vi "PhotonUtils_EstimateCameraToTargetTrans.vi"(10 "Yaw":T2={"VALUE"=0.0, "COS"=1.0, "SIN"=0.0} {"SIN" format="%13.4f"; "COS" format="%13.4f"; "VALUE" format="%13.4f"}, 11 "TargetDistance_Meters":dbl) -> (3 "CameraToTarget":T1 {"Y" format="%14.3f"; "X" format="%14.3f"})   [LabVIEW 2020, in "PhotonVisionLib.lvlib"]
doc: "Estimate the Translation2d of the target relative to the camera.\n \nInputs: \n - TargetDistance_Meters -- The distance to the target in meters.\n - Yaw -- The observed yaw of the target.\n\nOutputs:\n - CameraToTarget -- The target's camera-relative translation."
uses:
  PhotonVisionLib.lvlib
  <vilib>/Rock Robotics/WPI/ThirdParty/JAS_Junk/TrajLib/ROTATION2D.ctl
  <vilib>/Rock Robotics/WPI/ThirdParty/JAS_Junk/TrajLib/TRANSLATION2D.ctl
  <vilib>/Rock Robotics/WPI/ThirdParty/JAS_Junk/TrajLib/Trajectory_Library.lvlib
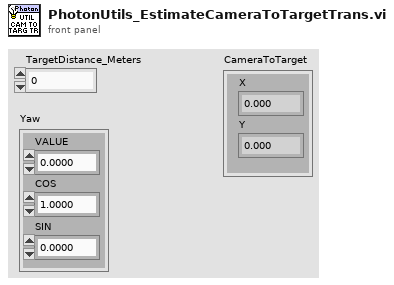
[diagram p1: front panel]
types:
  T1 = typedef "Trajectory_Library.lvlib/TRANSLATION2D.ctl" = cluster{"X":dbl, "Y":dbl}
  T2 = typedef "Trajectory_Library.lvlib/ROTATION2D.ctl" = cluster{"VALUE":dbl, "COS":dbl, "SIN":dbl}
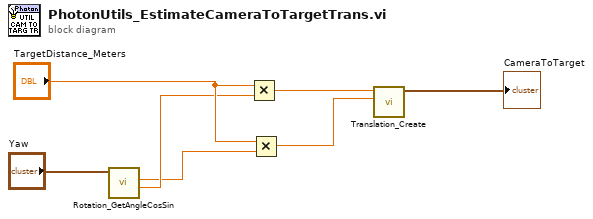
[diagram p0: block diagram]
diagram:
  n1 = call <vilib>:"Rotation_GetAngleCosSin.vi"("in ROTATION"="Yaw") -> ("Cosine"=w5:dbl, "Sine"=w4:dbl)  [unwired: 8 in, 1 out]
  n2 = Multiply(x="TargetDistance_Meters", y=w5) -> (x*y=w3:dbl)
  n3 = Multiply(x="TargetDistance_Meters", y=w4) -> (x*y=w2:dbl)
  n4 = call <vilib>:"Translation_Create.vi"("Y"=w2, "X"=w3) -> ("TRANSLATION"=→"CameraToTarget":T1)  [unwired: 9 in]
